vi "Create DataColumns by Names and Types.vi"(8 "error in (no error)":errorcluster caption="错误输入（无错误）", 10 "DataColunm Types":variant[](array[variant]), 11 "DataColumn Names":string[](array[string])) -> (0 "error out":errorcluster caption="错误输出", 3 "DataColumns":refnum<class "Data Column.lvclass">[](array[class]))   [LabVIEW 2012, in "Data Grid VIEW.lvlib" / "Data Column.lvclass"]
uses:
  Data Column.lvclass
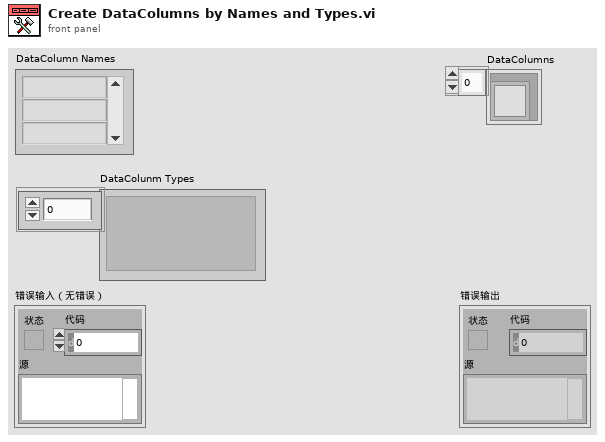
[diagram p1: front panel]
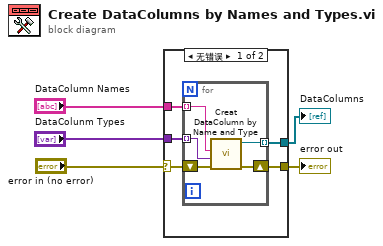
[diagram p0: block diagram]
diagram:
  n1 = case shown="无错误" "error in (no error)" {
    selector: "error in (no error)" -> [w8 w16]
    tunnel: [w6 w16] -> w4
    tunnel: "DataColumn Names" -> [w10 _]
    tunnel: "DataColunm Types" -> [w9 _]
    tunnel: [w7 _] -> w1
    frame No Error {
      n2 = for {
        tunnel: w10 -> [w15] mode=indexing
        tunnel: w9 -> [w14] mode=indexing
        shift-right: [w12] -> w6
        shift-left: w8 -> [w13]
        tunnel: [w11] -> w7 mode=indexing
        n3 = call "Creat DataColumn by Name and Type.vi"("error in (no error)"=w13, "anything"=w14, "columnName"=w15) -> ("error out"=w12:errorcluster, "Data Column 输出"=w11:refnum<class "Data Column.lvclass">)  [unwired: 7 in]
      }
    }
    frame Error {
    }
  }
  "error out" <- w4
  "DataColumns" <- w1
